vi "VirtualChannelTimerTracepoint.vi"(7 "service name":string, 8 "error in (no error)":errorcluster, 10 "Running Avg":dbl, 11 "Qbus in":refnum<class "Qbus.lvclass">) -> (0 "error out":errorcluster)   [LabVIEW 2017]
uses:
  <vilib>/addons/Qbus/Qbus.lvclass
  <vilib>/addons/TraceLogger/TraceLogger.lvlib
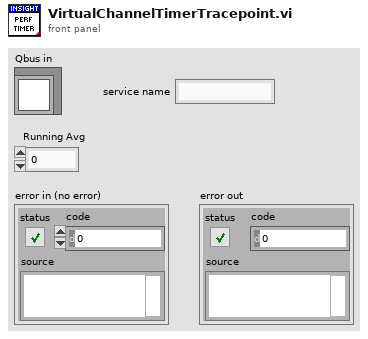
[diagram p1: front panel]
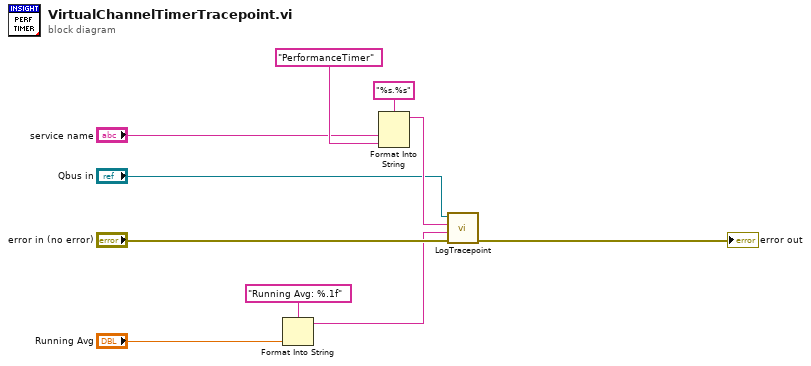
[diagram p0: block diagram]
diagram:
  n1 = Format Into String(format string="Running Avg: %.1f", "Running Avg") -> (resulting string=w1:string)  [unwired: 2 in, 1 out]
  n2 = Format Into String(format string="%s.%s", "service name", "PerformanceTimer" ("tracepoint")) -> (resulting string=w7:string)  [unwired: 2 in, 1 out]
  n3 = call <vilib>:"LogTracepoint.vi"("error in (no error)"="error in (no error)", "log string"=w1, "tracepoint"=w7, "qbus in"="Qbus in") -> ("error out"=→"error out":errorcluster)  [unwired: 6 in, 1 out]
